vi "AlGaInPAs_prep_run_cont_v04.vi"(2 "Debug Mode":bool, 3 "Elapsed Time(s)":dbl, 4 "State":enum16{"Edit", "Start", "Run", "End", "Idle"}(ring), 5 "Argument List In":string[](array[string])) -> (0 "Status Out":string, 1 "Argument List Out":string[](array[string]))   [LabVIEW 2011]
panel:
  out "total time":dbl
  out "is OK?":bool
  out "AsH3?":bool
  out "PH3?":bool
  out "In?":bool
  out "Ga?":bool
  out "Al?":bool
  in  "Prep As":bool caption="Pre-run"
  in  "Prep P":bool caption="Pre-run"
  in  "Prep In":bool caption="Pre-run"
  in  "Prep Ga":bool caption="Pre-run"
  in  "prep_time":dbl caption="pre-run time (s)"
  in  "Prep Al":bool caption="Pre-run"
  in  "Run As":bool caption="Run"
  in  "AsH3 Flow":dbl caption="AsH3 Flow (0-10 sccm)" format="%.2f"
  in  "P Flow":dbl caption="P Flow (0-100 sccm)" format="%.2f"
  in  "Run P":bool caption="Run"
  in  "In Flow":dbl caption="In Flow (0-100 sscm)" format="%.2f"
  in  "Run In":bool caption="Run"
  in  "Run Ga":bool caption="Run"
  in  "Ga Flow":dbl caption="Ga Flow (0-10 sscm)" format="%.2f"
  in  "Run Al":bool caption="Run"
  in  "Al Flow":dbl caption="Al Flow (0-100 sscm)" format="%.2f"
  in  "Cancel":bool
  in  "OK":bool
  out "tTotal(s) 2":dbl
  # "Add pre-run time to run time in editor."
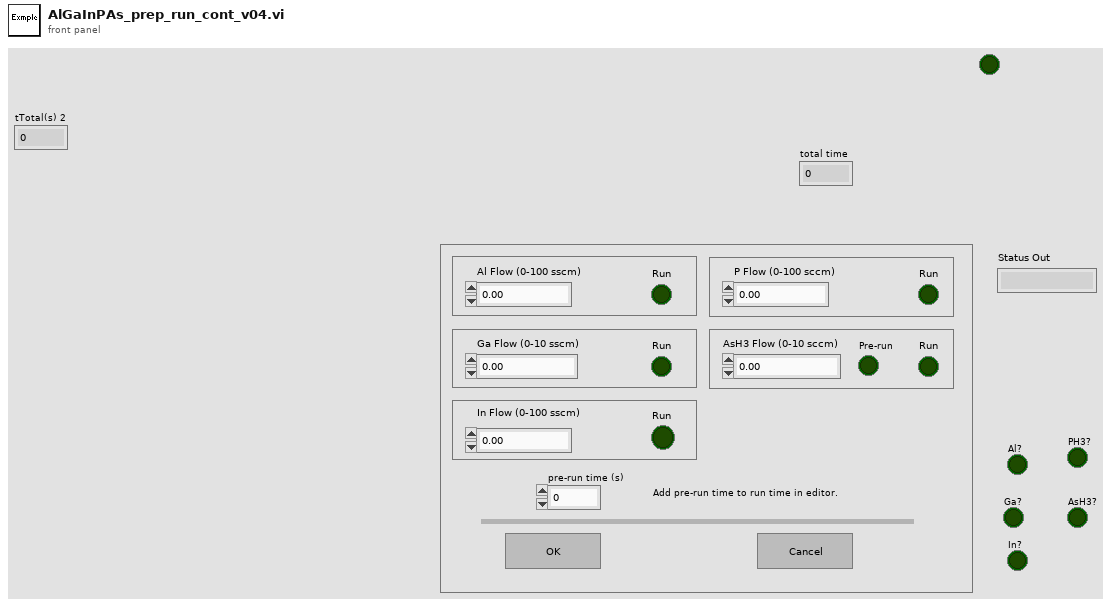
[diagram p1: front panel]
types:
  T1 = enum16{"Discrete", "Continuous", "Instantaneous"}
  T2 = enum32{"Invalid", "Default", "Floating", "Floating/Auto-Hide", "Modal"}
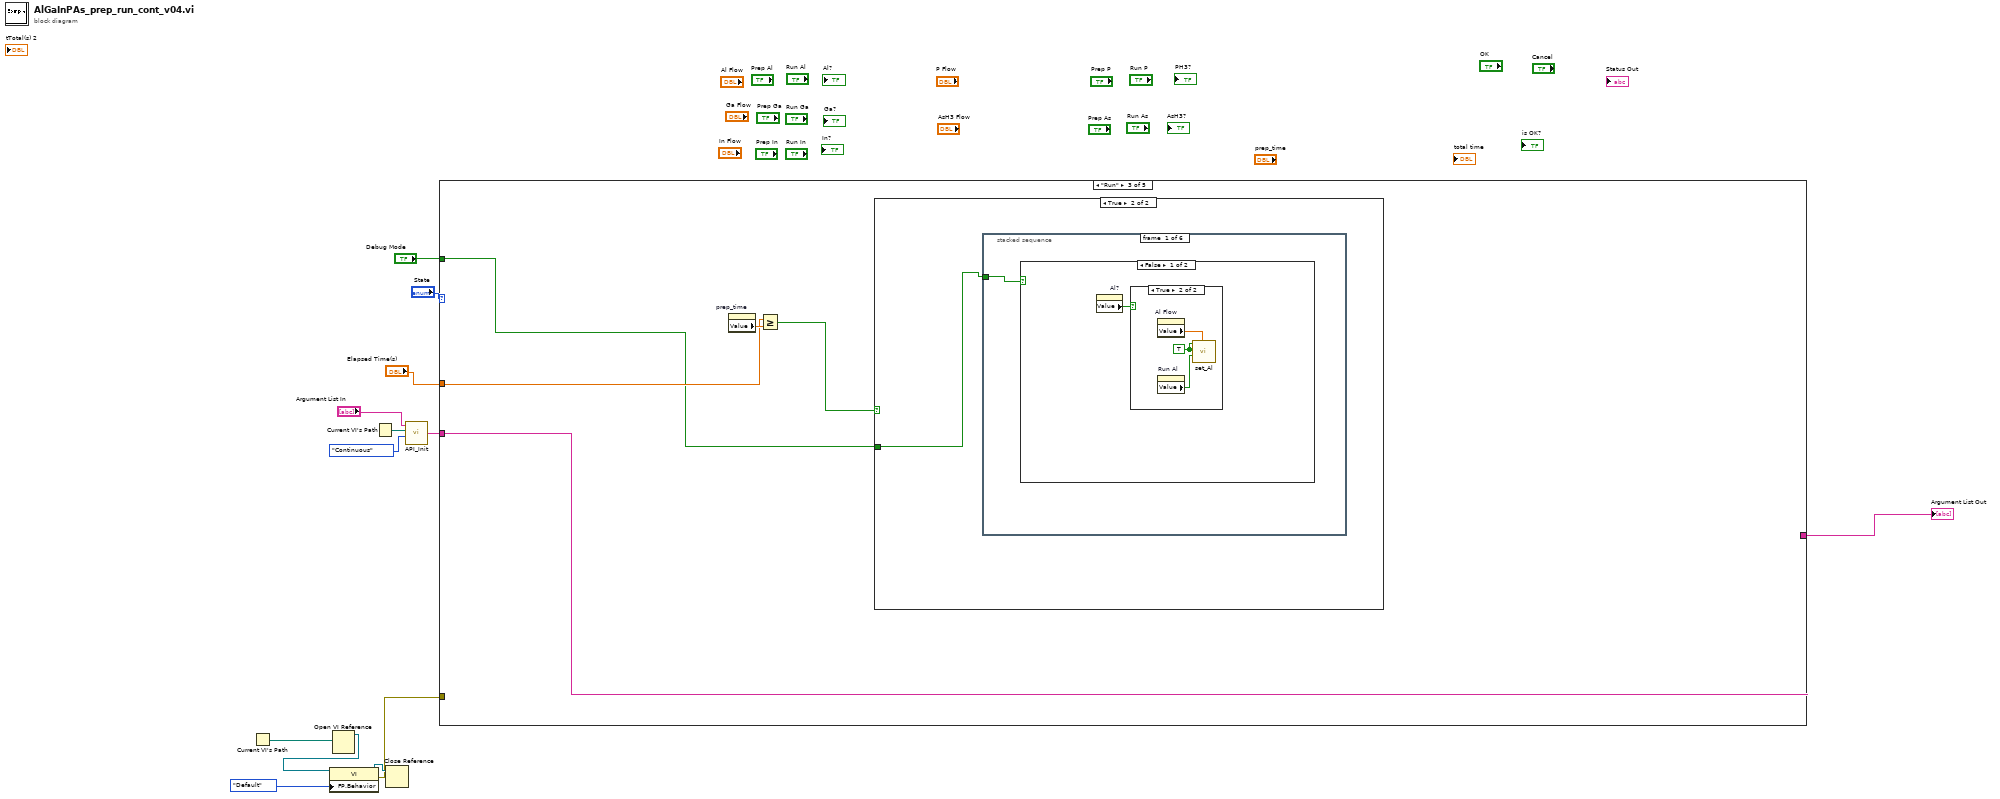
[diagram p0: block diagram]
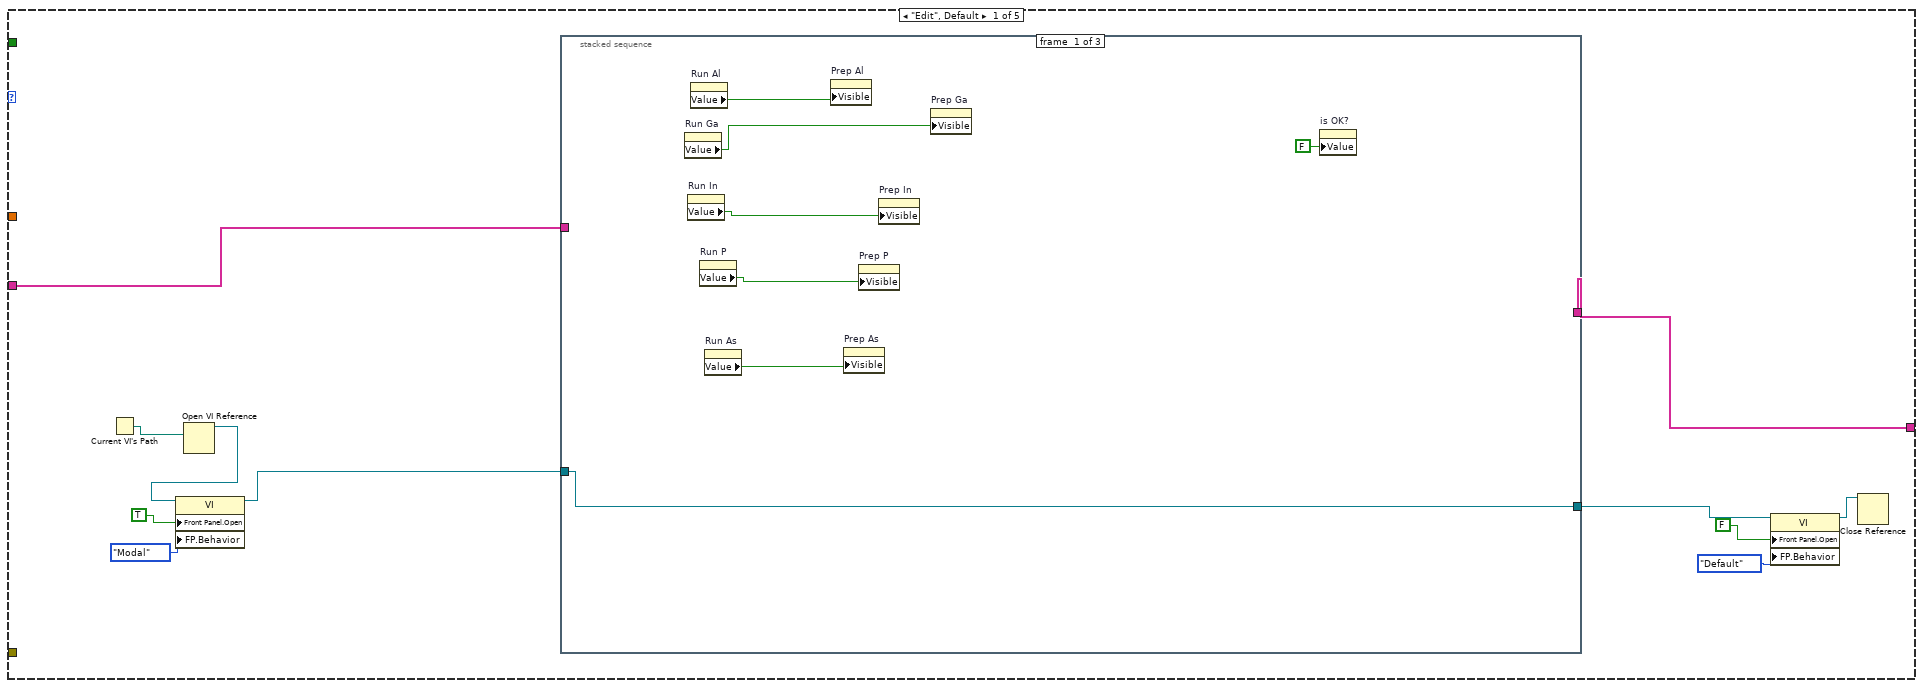
[diagram p2: hidden frame]
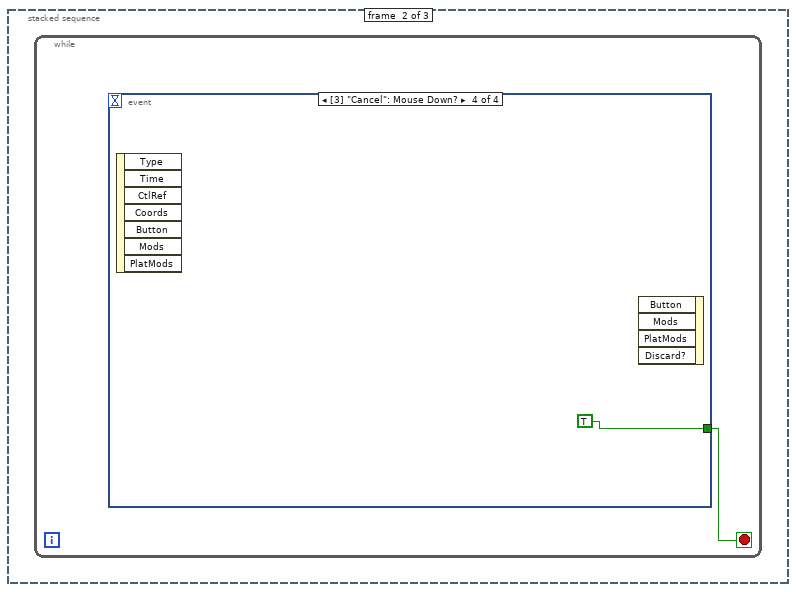
[diagram p3: hidden frame]
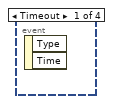
[diagram p4: hidden frame]
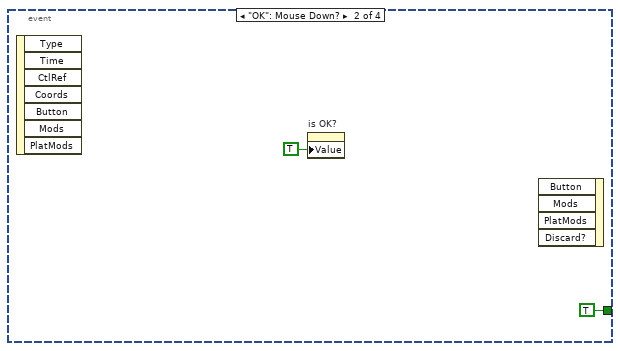
[diagram p5: hidden frame]
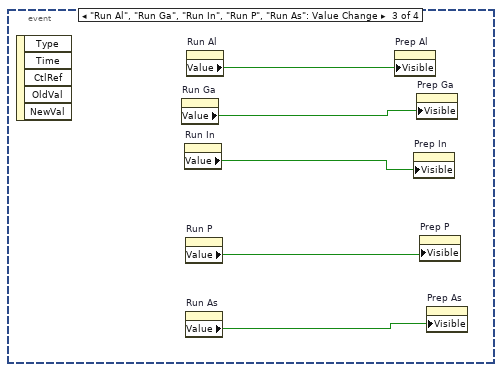
[diagram p6: hidden frame]
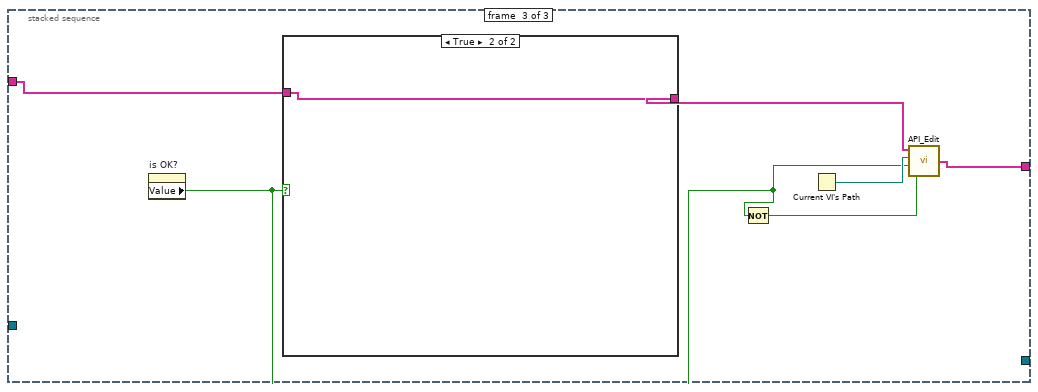
[diagram p7: hidden frame]
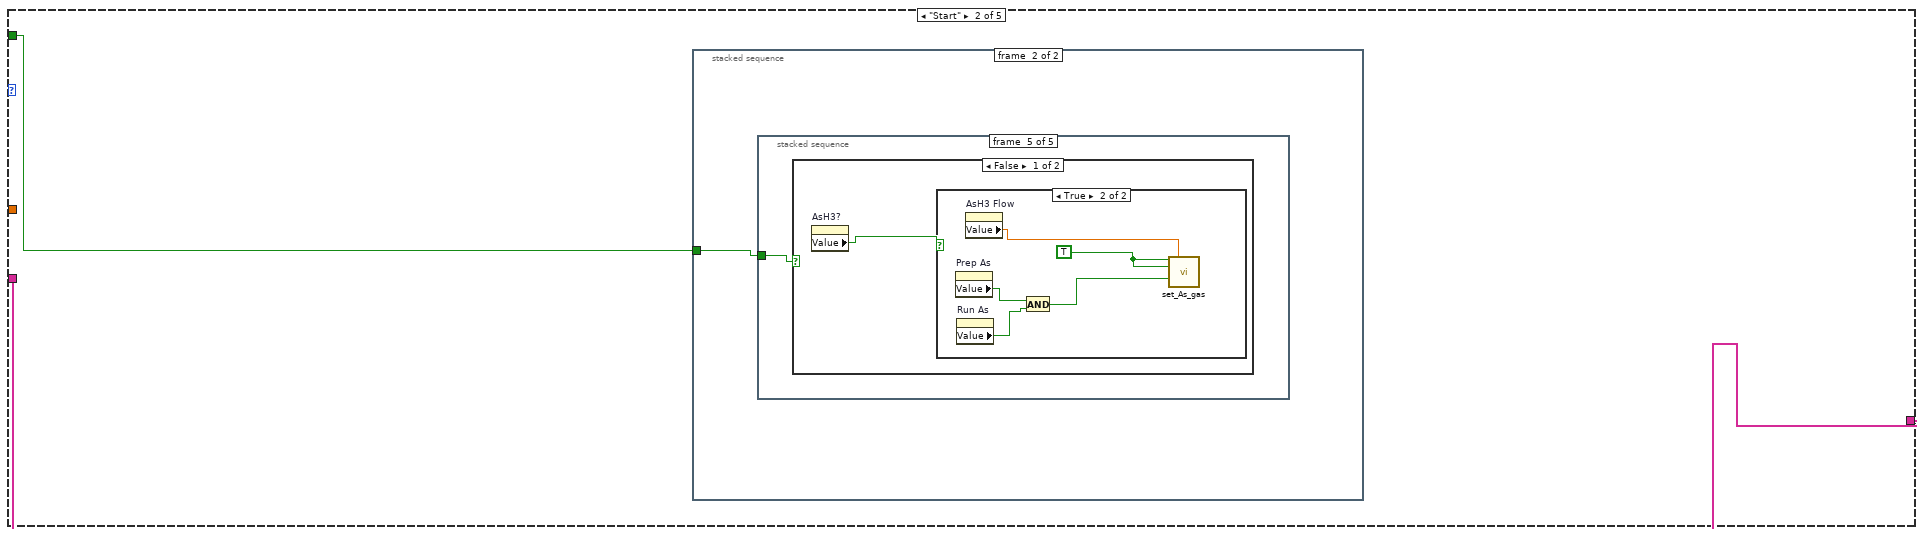
[diagram p9: hidden frame]
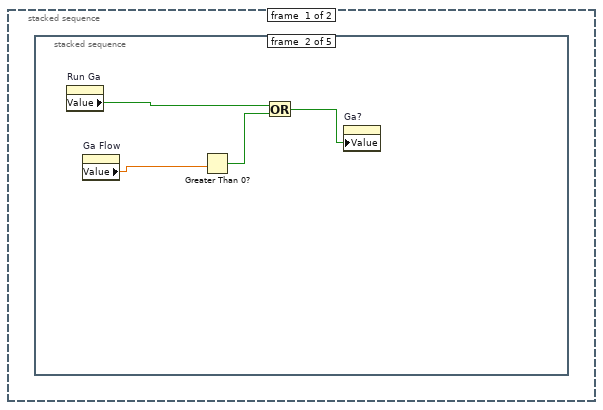
[diagram p10: hidden frame]
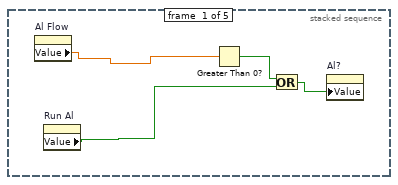
[diagram p11: hidden frame]
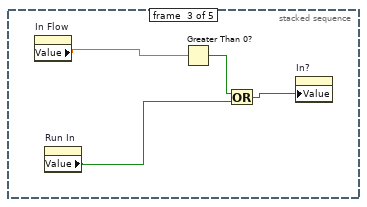
[diagram p12: hidden frame]
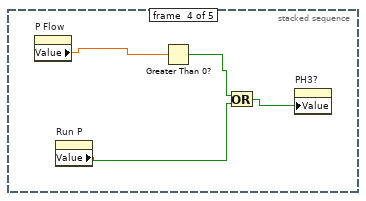
[diagram p13: hidden frame]
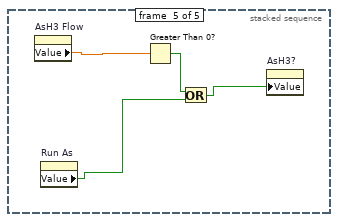
[diagram p14: hidden frame]
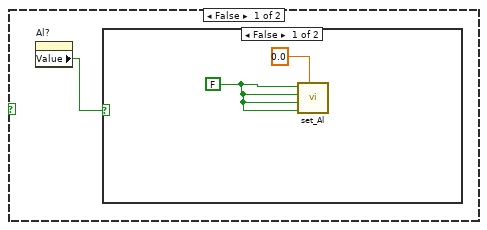
[diagram p16: hidden frame]
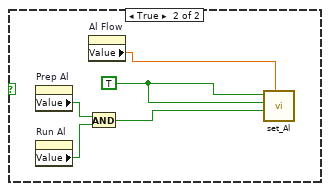
[diagram p17: hidden frame]
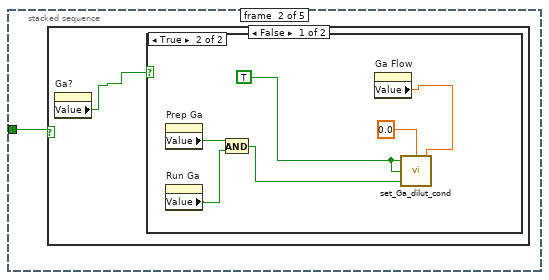
[diagram p18: hidden frame]
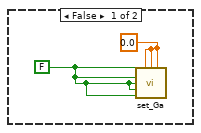
[diagram p19: hidden frame]
diagram:
  n1 = Current VI's Path() -> (path=w9:path)
  n2 = Open VI Reference(vi path=w9) -> (vi reference=w8:refnum<vi>)  [unwired: 1 in, 5 out]
  n3 = property class="VI"(reference=w8, "FP.Behavior"=T2."Default" ("Front Panel Window:Behavior")) -> (reference out=w6:refnum<vi>, error out=w5:errorcluster)  [unwired: 1 in]
  n4 = Current VI's Path() -> (path=w4:path)
  n5 = Close Reference(reference=w6) -> ()  [unwired: 1 in, 1 out]
  n6 = call "API_Init.vi"("API Mode"=T1."Continuous", "VI Path"=w4, "Argument List In"="Argument List In") -> ("Argument List Out"=w1:string[])  [unwired: 1 in]
  n7 = case shown="\"Run\"" "State" {
    tunnel: "Debug Mode" -> [_ w49 w119 _ _]
    tunnel: "Elapsed Time(s)" -> [_ _ w120 _ _]
    tunnel: w1 -> [w15 w50 w122 w162 w163]
    tunnel: [w14 w50 w122 w162 w163] -> w10
    tunnel: w5 -> [_ _ _ _ _]
    frame "Edit", Default {
      n8 = Current VI's Path() -> (path=w20:path)
      n9 = Open VI Reference(vi path=w20) -> (vi reference=w19:refnum<vi>)  [unwired: 1 in, 5 out]
      n10 = property class="VI"(reference=w19, "Front Panel.Open"=TRUE ("Front Panel Window:Open"), "FP.Behavior"=T2."Modal" ("Front Panel Window:Behavior")) -> (reference out=w18:refnum<vi>)  [unwired: 1 in, 1 out]
      n11 = stacked-sequence {
        tunnel: w15 -> [_ _ w44]
        tunnel: w18 -> [w31 _ _]
        tunnel: [w31 _ _] -> w22
        tunnel: [_ _ w42] -> w14
        frame #0 {
          n12 = property on="Run Ga" class="Bool (strict)"() -> ("Value"=w28:bool)  [unwired: 2 in, 2 out]
          n13 = property on="Run In" class="Bool (strict)"() -> ("Value"=w27:bool)  [unwired: 2 in, 2 out]
          n14 = property on="Run Al" class="Bool (strict)"() -> ("Value"=w29:bool)  [unwired: 2 in, 2 out]
          n15 = property on="Run P" class="Bool (strict)"() -> ("Value"=w26:bool)  [unwired: 2 in, 2 out]
          n16 = property on="Run As" class="Bool (strict)"() -> ("Value"=w25:bool)  [unwired: 2 in, 2 out]
          n17 = property on="Prep Al" class="Bool (strict)"("Visible"=w29) -> ()  [unwired: 2 in, 2 out]
          n18 = property on="Prep As" class="Bool (strict)"("Visible"=w25) -> ()  [unwired: 2 in, 2 out]
          n19 = property on="Prep P" class="Bool (strict)"("Visible"=w26) -> ()  [unwired: 2 in, 2 out]
          n20 = property on="Prep In" class="Bool (strict)"("Visible"=w27) -> ()  [unwired: 2 in, 2 out]
          n21 = property on="Prep Ga" class="Bool (strict)"("Visible"=w28) -> ()  [unwired: 2 in, 2 out]
          n22 = property on="is OK?" class="Bool (strict)"("Value"=FALSE ("is OK?")) -> ()  [unwired: 2 in, 2 out]
        }
        frame #1 {
          n23 = while {
            stop <- w32 stop-if-true
            n24 = event shown="[3] \"Cancel\": Mouse Down?" {
              selector: _ -> [_ _ _ _]
              dyn-events: _ -> [_ _ _ _]
              timeout: _ -> [_ _ _ _]
              tunnel: [_ TRUE _ TRUE] -> w32
              event Timeout {
                n25 = event-data() -> ()  [unwired: 1 in, 2 out]
              }
              event "OK": Mouse Down? {
                n26 = event-data() -> ()  [unwired: 1 in, 7 out]
                n27 = property on="is OK?" class="Bool (strict)"("Value"=TRUE ("is OK?")) -> ()  [unwired: 2 in, 2 out]
                n28 = event-data() -> ()  [unwired: 5 in, 1 out]
              }
              event "Run Al", "Run Ga", "Run In", "Run P", "Run As": Value Change {
                n29 = event-data() -> ()  [unwired: 1 in, 5 out]
                n30 = property on="Run Ga" class="Bool (strict)"() -> ("Value"=w38:bool)  [unwired: 2 in, 2 out]
                n31 = property on="Run In" class="Bool (strict)"() -> ("Value"=w37:bool)  [unwired: 2 in, 2 out]
                n32 = property on="Run P" class="Bool (strict)"() -> ("Value"=w36:bool)  [unwired: 2 in, 2 out]
                n33 = property on="Run As" class="Bool (strict)"() -> ("Value"=w35:bool)  [unwired: 2 in, 2 out]
                n34 = property on="Run Al" class="Bool (strict)"() -> ("Value"=w39:bool)  [unwired: 2 in, 2 out]
                n35 = property on="Prep Al" class="Bool (strict)"("Visible"=w39) -> ()  [unwired: 2 in, 2 out]
                n36 = property on="Prep In" class="Bool (strict)"("Visible"=w37) -> ()  [unwired: 2 in, 2 out]
                n37 = property on="Prep Ga" class="Bool (strict)"("Visible"=w38) -> ()  [unwired: 2 in, 2 out]
                n38 = property on="Prep P" class="Bool (strict)"("Visible"=w36) -> ()  [unwired: 2 in, 2 out]
                n39 = property on="Prep As" class="Bool (strict)"("Visible"=w35) -> ()  [unwired: 2 in, 2 out]
              }
              event "Cancel": Mouse Down? {
                n40 = event-data() -> ()  [unwired: 1 in, 7 out]
                n41 = event-data() -> ()  [unwired: 5 in, 1 out]
              }
            }
          }
        }
        frame #2 {
          n42 = property on="is OK?" class="Bool (strict)"() -> ("Value"=w41:bool)  [unwired: 2 in, 2 out]
          n43 = case shown="True" w41 {
            tunnel: w44 -> [w47 w48]
            tunnel: [w47 w48] -> w43
            frame False {
            }
            frame True {
            }
          }
          n44 = Not(x=w41) -> (.not. x?=w46:bool)
          n45 = Current VI's Path() -> (path=w45:path)
          n46 = call "API_Edit.vi"("Cancel"=w46, "OK"=w41, "VI Path"=w45, "Argument List In"=w43) -> ("Argument List Out"=w42:string[])
        }
      }
      n47 = property class="VI"(reference=w22, "Front Panel.Open"=FALSE ("Front Panel Window:Open"), "FP.Behavior"=T2."Default" ("Front Panel Window:Behavior")) -> (reference out=w23:refnum<vi>)  [unwired: 1 in, 1 out]
      n48 = Close Reference(reference=w23) -> ()  [unwired: 1 in, 1 out]
    }
    frame "Start" {
      n49 = stacked-sequence {
        tunnel: w49 -> [_ w71]
        frame #0 {
          n50 = stacked-sequence {
            frame #0 {
              n51 = property on="Al Flow" class="DigNum (strict)"() -> ("Value"=w53:dbl)  [unwired: 2 in, 2 out]
              n52 = property on="Run Al" class="Bool (strict)"() -> ("Value"=w52:bool)  [unwired: 2 in, 2 out]
              n53 = Greater Than 0?(x=w53) -> (x > 0?=w54:bool)
              n54 = Or(x=w54, y=w52) -> (x .or. y?=w51:bool)
              n55 = property on="Al?" class="Bool (strict)"("Value"=w51) -> ()  [unwired: 2 in, 2 out]
            }
            frame #1 {
              n56 = property on="Run Ga" class="Bool (strict)"() -> ("Value"=w56:bool)  [unwired: 2 in, 2 out]
              n57 = property on="Ga Flow" class="DigNum (strict)"() -> ("Value"=w57:dbl)  [unwired: 2 in, 2 out]
              n58 = Greater Than 0?(x=w57) -> (x > 0?=w58:bool)
              n59 = Or(x=w56, y=w58) -> (x .or. y?=w55:bool)
              n60 = property on="Ga?" class="Bool (strict)"("Value"=w55) -> ()  [unwired: 2 in, 2 out]
            }
            frame #2 {
              n61 = property on="In Flow" class="DigNum (strict)"() -> ("Value"=w60:dbl)  [unwired: 2 in, 2 out]
              n62 = property on="Run In" class="Bool (strict)"() -> ("Value"=w61:bool)  [unwired: 2 in, 2 out]
              n63 = Greater Than 0?(x=w60) -> (x > 0?=w62:bool)
              n64 = Or(x=w62, y=w61) -> (x .or. y?=w59:bool)
              n65 = property on="In?" class="Bool (strict)"("Value"=w59) -> ()  [unwired: 2 in, 2 out]
            }
            frame #3 {
              n66 = property on="P Flow" class="DigNum (strict)"() -> ("Value"=w65:dbl)  [unwired: 2 in, 2 out]
              n67 = property on="Run P" class="Bool (strict)"() -> ("Value"=w64:bool)  [unwired: 2 in, 2 out]
              n68 = Greater Than 0?(x=w65) -> (x > 0?=w66:bool)
              n69 = Or(x=w66, y=w64) -> (x .or. y?=w63:bool)
              n70 = property on="PH3?" class="Bool (strict)"("Value"=w63) -> ()  [unwired: 2 in, 2 out]
            }
            frame #4 {
              n71 = property on="AsH3 Flow" class="DigNum (strict)"() -> ("Value"=w69:dbl)  [unwired: 2 in, 2 out]
              n72 = property on="Run As" class="Bool (strict)"() -> ("Value"=w68:bool)  [unwired: 2 in, 2 out]
              n73 = Greater Than 0?(x=w69) -> (x > 0?=w70:bool)
              n74 = Or(x=w70, y=w68) -> (x .or. y?=w67:bool)
              n75 = property on="AsH3?" class="Bool (strict)"("Value"=w67) -> ()  [unwired: 2 in, 2 out]
            }
          }
        }
        frame #1 {
          n76 = stacked-sequence {
            tunnel: w71 -> [w72 w81 w91 w100 w109]
            frame #0 {
              n77 = case shown="True" w72 {
                frame False {
                  n78 = property on="Al?" class="Bool (strict)"() -> ("Value"=w73:bool)  [unwired: 2 in, 2 out]
                  n79 = case shown="False" w73 {
                    frame False {
                      w74 = FALSE ("Al Active")
                      n80 = call "set_Al.vi"("Aluminum Flow"=0.0, "Al Remote"=w74, "Al Run"=w74, "Al Bubbler"=w74, "Al Active"=w74) -> ()  [unwired: 5 out]
                    }
                    frame True {
                      w80 = TRUE ("Al Active")
                      n81 = property on="Prep Al" class="Bool (strict)"() -> ("Value"=w78:bool)  [unwired: 2 in, 2 out]
                      n82 = property on="Run Al" class="Bool (strict)"() -> ("Value"=w77:bool)  [unwired: 2 in, 2 out]
                      n83 = property on="Al Flow" class="DigNum (strict)"() -> ("Value"=w79:dbl)  [unwired: 2 in, 2 out]
                      n84 = And(x=w78, y=w77) -> (x .and. y?=w76:bool)
                      n85 = call "set_Al.vi"("Aluminum Flow"=w79, "Al Run"=w76, "Al Bubbler"=w80, "Al Active"=w80) -> ()  [unwired: 1 in, 5 out]
                    }
                  }
                }
                frame True {
                }
              }
            }
            frame #1 {
              n86 = case shown="False" w81 {
                frame False {
                  n87 = property on="Ga?" class="Bool (strict)"() -> ("Value"=w82:bool)  [unwired: 2 in, 2 out]
                  n88 = case shown="True" w82 {
                    frame False {
                      w84 = FALSE ("Ga Active")
                      w83 = 0.0 ("Ga Flow 1")
                      n89 = call "set_Ga.vi"("Ga Active"=w84, "Ga Flow 3"=w83, "Ga Flow 2"=w83, "Ga Flow 1"=w83, "Ga Bubbler"=w84, "Ga H2 Dilute"=w84, "Ga Run"=w84, "Ga Remote"=w84) -> ()  [unwired: 8 out]
                    }
                    frame True {
                      w90 = TRUE ("Ga Active")
                      n90 = property on="Prep Ga" class="Bool (strict)"() -> ("Value"=w87:bool)  [unwired: 2 in, 2 out]
                      n91 = property on="Run Ga" class="Bool (strict)"() -> ("Value"=w86:bool)  [unwired: 2 in, 2 out]
                      n92 = And(x=w87, y=w86) -> (x .and. y?=w85:bool)
                      n93 = property on="Ga Flow" class="DigNum (strict)"() -> ("Value"=w88:dbl)  [unwired: 2 in, 2 out]
                      n94 = call "set_Ga_dilut_cond.vi"("Ga flow (0-10 sccm)"=w88, "fDilution"=0.0, "Run"=w85, "Bubbler In"=w90, "Active"=w90) -> ()
                    }
                  }
                }
                frame True {
                }
              }
            }
            frame #2 {
              n95 = case shown="False" w91 {
                frame False {
                  n96 = property on="In?" class="Bool (strict)"() -> ("Value"=w92:bool)  [unwired: 2 in, 2 out]
                  n97 = case shown="True" w92 {
                    frame False {
                      w94 = FALSE ("In Remote")
                      n98 = call "set_In.vi"("Indium Flow"=0.0, "In Remote"=w94, "In Run"=w94, "In Bubbler"=w94, "In Active"=w94) -> ()  [unwired: 5 out]
                    }
                    frame True {
                      w99 = TRUE ("In Run")
                      n99 = property on="Run In" class="Bool (strict)"() -> ("Value"=w96:bool)  [unwired: 2 in, 2 out]
                      n100 = property on="Prep In" class="Bool (strict)"() -> ("Value"=w97:bool)  [unwired: 2 in, 2 out]
                      n101 = And(x=w97, y=w96) -> (x .and. y?=w95:bool)
                      n102 = property on="In Flow" class="DigNum (strict)"() -> ("Value"=w98:dbl)  [unwired: 2 in, 2 out]
                      n103 = call "set_In.vi"("Indium Flow"=w98, "In Run"=w95, "In Bubbler"=w99, "In Active"=w99) -> ()  [unwired: 1 in, 5 out]
                    }
                  }
                }
                frame True {
                }
              }
            }
            frame #3 {
              n104 = case shown="False" w100 {
                frame False {
                  n105 = property on="PH3?" class="Bool (strict)"() -> ("Value"=w101:bool)  [unwired: 2 in, 2 out]
                  n106 = case shown="True" w101 {
                    frame False {
                      w102 = FALSE ("P_Gas Active")
                      n107 = call "set_P_gas.vi"("P_Gas Active"=w102, "P_Gas Flow"=0.0, "P_Gas In"=w102, "P_Gas H2 In"=w102, "P_Gas Run"=w102, "P_Gas Remote"=w102) -> ()  [unwired: 10 out]
                    }
                    frame True {
                      w108 = TRUE ("P_Gas Active")
                      n108 = property on="P Flow" class="DigNum (strict)"() -> ("Value"=w107:dbl)  [unwired: 2 in, 2 out]
                      n109 = property on="Prep P" class="Bool (strict)"() -> ("Value"=w106:bool)  [unwired: 2 in, 2 out]
                      n110 = property on="Run P" class="Bool (strict)"() -> ("Value"=w105:bool)  [unwired: 2 in, 2 out]
                      n111 = And(x=w106, y=w105) -> (x .and. y?=w104:bool)
                      n112 = call "set_P_gas.vi"("P_Gas Active"=w108, "P_Gas Flow"=w107, "P_Gas In"=w108, "P_Gas Run"=w104) -> ()  [unwired: 2 in, 10 out]
                    }
                  }
                }
                frame True {
                }
              }
            }
            frame #4 {
              n113 = case shown="False" w109 {
                frame False {
                  n114 = property on="AsH3?" class="Bool (strict)"() -> ("Value"=w110:bool)  [unwired: 2 in, 2 out]
                  n115 = case shown="True" w110 {
                    frame False {
                      w111 = FALSE ("As_Gas Active")
                      n116 = call "set_As_gas.vi"("As_Gas Active"=w111, "As_Gas Flow"=0.0, "As_Gas In"=w111, "As_Gas H2"=w111, "As_Gas Run"=w111, "As_Gas Remote"=w111) -> ()  [unwired: 10 in]
                    }
                    frame True {
                      w117 = TRUE ("As_Gas Active")
                      n117 = property on="Prep As" class="Bool (strict)"() -> ("Value"=w114:bool)  [unwired: 2 in, 2 out]
                      n118 = property on="Run As" class="Bool (strict)"() -> ("Value"=w115:bool)  [unwired: 2 in, 2 out]
                      n119 = property on="AsH3 Flow" class="DigNum (strict)"() -> ("Value"=w116:dbl)  [unwired: 2 in, 2 out]
                      n120 = And(x=w114, y=w115) -> (x .and. y?=w113:bool)
                      n121 = call "set_As_gas.vi"("As_Gas Active"=w117, "As_Gas Flow"=w116, "As_Gas In"=w117, "As_Gas Run"=w113) -> ()  [unwired: 12 in]
                    }
                  }
                }
                frame True {
                }
              }
            }
          }
        }
      }
    }
    frame "Run" {
      n122 = property on="prep_time" class="DigNum (strict)"() -> ("Value"=w121:dbl)  [unwired: 2 in, 2 out]
      n123 = Greater Or Equal?(x=w120, y=w121) -> (x >= y?=w118:bool)
      n124 = case shown="True" w118 {
        tunnel: w119 -> [_ w124]
        frame False {
          n125 = property on="Status Out" class="Str"("Value"="pre-run" ("Status Out")) -> ()  [unwired: 2 in, 2 out]
        }
        frame True {
          n126 = stacked-sequence {
            tunnel: w124 -> [w125 w132 w140 w147 w154 _]
            frame #0 {
              n127 = case shown="False" w125 {
                frame False {
                  n128 = property on="Al?" class="Bool (strict)"() -> ("Value"=w126:bool)  [unwired: 2 in, 2 out]
                  n129 = case shown="True" w126 {
                    frame False {
                      w127 = FALSE ("Al Active")
                      n130 = call "set_Al.vi"("Aluminum Flow"=0.0, "Al Remote"=w127, "Al Run"=w127, "Al Bubbler"=w127, "Al Active"=w127) -> ()  [unwired: 5 out]
                    }
                    frame True {
                      w131 = TRUE ("Al Active")
                      n131 = property on="Al Flow" class="DigNum (strict)"() -> ("Value"=w130:dbl)  [unwired: 2 in, 2 out]
                      n132 = property on="Run Al" class="Bool (strict)"() -> ("Value"=w129:bool)  [unwired: 2 in, 2 out]
                      n133 = call "set_Al.vi"("Aluminum Flow"=w130, "Al Run"=w129, "Al Bubbler"=w131, "Al Active"=w131) -> ()  [unwired: 1 in, 5 out]
                    }
                  }
                }
                frame True {
                }
              }
            }
            frame #1 {
              n134 = case shown="False" w132 {
                frame False {
                  n135 = property on="Ga?" class="Bool (strict)"() -> ("Value"=w133:bool)  [unwired: 2 in, 2 out]
                  n136 = case shown="False" w133 {
                    frame False {
                      w135 = FALSE ("Ga Active")
                      w134 = 0.0 ("Ga Flow 1")
                      n137 = call "set_Ga.vi"("Ga Active"=w135, "Ga Flow 3"=w134, "Ga Flow 2"=w134, "Ga Flow 1"=w134, "Ga Bubbler"=w135, "Ga H2 Dilute"=w135, "Ga Run"=w135, "Ga Remote"=w135) -> ()  [unwired: 8 out]
                    }
                    frame True {
                      w139 = TRUE ("Ga Active")
                      n138 = property on="Ga Flow" class="DigNum (strict)"() -> ("Value"=w136:dbl)  [unwired: 2 in, 2 out]
                      n139 = property on="Run Ga" class="Bool (strict)"() -> ("Value"=w137:bool)  [unwired: 2 in, 2 out]
                      n140 = call "set_Ga_dilut_cond.vi"("Ga flow (0-10 sccm)"=w136, "fDilution"=0.0, "Run"=w137, "Bubbler In"=w139, "Active"=w139) -> ()
                    }
                  }
                }
                frame True {
                }
              }
            }
            frame #2 {
              n141 = case shown="False" w140 {
                frame False {
                  n142 = property on="In?" class="Bool (strict)"() -> ("Value"=w141:bool)  [unwired: 2 in, 2 out]
                  n143 = case shown="True" w141 {
                    frame False {
                      w143 = FALSE ("In Remote")
                      n144 = call "set_In.vi"("Indium Flow"=0.0, "In Remote"=w143, "In Run"=w143, "In Bubbler"=w143, "In Active"=w143) -> ()  [unwired: 5 out]
                    }
                    frame True {
                      w146 = TRUE ("In Run")
                      n145 = property on="Run In" class="Bool (strict)"() -> ("Value"=w144:bool)  [unwired: 2 in, 2 out]
                      n146 = property on="In Flow" class="DigNum (strict)"() -> ("Value"=w145:dbl)  [unwired: 2 in, 2 out]
                      n147 = call "set_In.vi"("Indium Flow"=w145, "In Run"=w144, "In Bubbler"=w146, "In Active"=w146) -> ()  [unwired: 1 in, 5 out]
                    }
                  }
                }
                frame True {
                }
              }
            }
            frame #3 {
              n148 = case shown="False" w147 {
                frame False {
                  n149 = property on="PH3?" class="Bool (strict)"() -> ("Value"=w148:bool)  [unwired: 2 in, 2 out]
                  n150 = case shown="False" w148 {
                    frame False {
                      w149 = FALSE ("P_Gas Active")
                      n151 = call "set_P_gas.vi"("P_Gas Active"=w149, "P_Gas Flow"=0.0, "P_Gas In"=w149, "P_Gas H2 In"=w149, "P_Gas Run"=w149, "P_Gas Remote"=w149) -> ()  [unwired: 10 out]
                    }
                    frame True {
                      w153 = TRUE ("P_Gas Active")
                      n152 = property on="P Flow" class="DigNum (strict)"() -> ("Value"=w152:dbl)  [unwired: 2 in, 2 out]
                      n153 = property on="Run P" class="Bool (strict)"() -> ("Value"=w151:bool)  [unwired: 2 in, 2 out]
                      n154 = call "set_P_gas.vi"("P_Gas Active"=w153, "P_Gas Flow"=w152, "P_Gas In"=w153, "P_Gas Run"=w151) -> ()  [unwired: 2 in, 10 out]
                    }
                  }
                }
                frame True {
                }
              }
            }
            frame #4 {
              n155 = case shown="False" w154 {
                frame False {
                  n156 = property on="AsH3?" class="Bool (strict)"() -> ("Value"=w155:bool)  [unwired: 2 in, 2 out]
                  n157 = case shown="False" w155 {
                    frame False {
                      w156 = FALSE ("As_Gas Active")
                      n158 = call "set_As_gas.vi"("As_Gas Active"=w156, "As_Gas Flow"=0.0, "As_Gas In"=w156, "As_Gas H2"=w156, "As_Gas Run"=w156, "As_Gas Remote"=w156) -> ()  [unwired: 10 in]
                    }
                    frame True {
                      w159 = TRUE ("As_Gas Active")
                      n159 = property on="Run As" class="Bool (strict)"() -> ("Value"=w158:bool)  [unwired: 2 in, 2 out]
                      n160 = property on="AsH3 Flow" class="DigNum (strict)"() -> ("Value"=w160:dbl)  [unwired: 2 in, 2 out]
                      n161 = call "set_As_gas.vi"("As_Gas Active"=w159, "As_Gas Flow"=w160, "As_Gas In"=w159, "As_Gas Run"=w158) -> ()  [unwired: 12 in]
                    }
                  }
                }
                frame True {
                }
              }
            }
            frame #5 {
              n162 = property on="Status Out" class="Str"("Value"="run started" ("Status Out")) -> ()  [unwired: 2 in, 2 out]
            }
          }
        }
      }
    }
    frame "End" {
    }
    frame "Idle" {
    }
  }
  "Argument List Out" <- w10
